vi "Control_Sensing_Sep.vi"() -> ()   [LabVIEW 2019]
uses:
  Control 1.ctl
  <vilib>/myRIO/Instrument Drivers/Onboard IO/I2C/typedefs/I2C User Configuration.ctl
  <vilib>/myRIO/Instrument Drivers/Onboard IO/I2C/typedefs/I2C Transfer Rate.ctl
  <vilib>/myRIO/Instrument Drivers/Onboard IO/I2C/typedefs/I2C Reference.ctl
  <vilib>/myRIO/Common/Instrument Driver Framework/Utilities/typedefs/myRIO Generic Hardware Reference.ctl
  <vilib>/myRIO/Common/Instrument Driver Framework/Utilities/typedefs/Hardware Version Enum.ctl
  <vilib>/myRIO/Common/Instrument Driver Framework/Utilities/typedefs/myRIO v1.0 Reference.ctl
  <vilib>/myRIO/Common/Instrument Driver Framework/Utilities/typedefs/Generic FPGA Reference.ctl
  <vilib>/myRIO/Common/Instrument Driver Framework/myRIO v1.0/I2C/typedefs/I2C Channels Enum.ctl
  <vilib>/myRIO/Instrument Drivers/Onboard IO/I2C/typedefs/I2C Configuration.ctl
  <vilib>/userDefined/High Color/nirio_resource_hc.ctl
  <vilib>/myRIO/Instrument Drivers/Onboard IO/AI/typedefs/AI Reference.ctl
  <vilib>/myRIO/Common/Instrument Driver Framework/myRIO v1.0/AI/typedefs/AI Channels List.ctl
  <vilib>/myRIO/Common/Instrument Driver Framework/myRIO v1.0/AI/typedefs/AI Channels Enum.ctl
  <vilib>/myRIO/Common/Instrument Driver Framework/Utilities/typedefs/Analog Scaling Constants List.ctl
  <vilib>/myRIO/Common/Instrument Driver Framework/Utilities/typedefs/Analog Scaling Constants.ctl
  <vilib>/myRIO/Instrument Drivers/Onboard IO/DIO/typedefs/DIO Reference.ctl
  <vilib>/myRIO/Common/Instrument Driver Framework/myRIO v1.0/DIO/typedefs/DIO Channels List.ctl
  <vilib>/myRIO/Common/Instrument Driver Framework/myRIO v1.0/DIO/typedefs/DIO Channels Enum.ctl
  <vilib>/myRIO/Instrument Drivers/Onboard IO/PWM/typedefs/PWM Reference.ctl
  <vilib>/myRIO/Common/Instrument Driver Framework/myRIO v1.0/PWM/typedefs/PWM Channels Enum.ctl
  <vilib>/myRIO/Instrument Drivers/Onboard IO/PWM/typedefs/PWM Configuration.ctl
  <vilib>/myRIO/Common/Instrument Driver Framework/Utilities/vis/Is FPGA Ref Available.vi
  <vilib>/myRIO/Common/Instrument Driver Framework/myRIO v1.0/I2C/vis/myRIO v1.1 Open I2C.vi
  <vilib>/myRIO/Instrument Drivers/Onboard IO/I2C/vis/Configure.vi
  <vilib>/myRIO/Instrument Drivers/Onboard IO/I2C/vis/Write.vi
  <vilib>/myRIO/Common/Instrument Driver Framework/myRIO v1.0/DIO/vis/myRIO v1.1 Open DIO.vi
  <vilib>/myRIO/Instrument Drivers/Onboard IO/DIO/vis/Read.vi
  <vilib>/myRIO/Common/Instrument Driver Framework/myRIO v1.0/AI/vis/myRIO v1.1 Open AI.vi
  <vilib>/myRIO/Instrument Drivers/Onboard IO/AI/vis/Read.vi
  <vilib>/myRIO/Instrument Drivers/Onboard IO/DIO/vis/Write.vi
  <vilib>/myRIO/Common/Instrument Driver Framework/myRIO v1.0/PWM/vis/myRIO v1.1 Open PWM.vi
  <vilib>/myRIO/Instrument Drivers/Onboard IO/PWM/vis/Set Duty Cycle and Frequency.vi
  <vilib>/myRIO/Instrument Drivers/Onboard IO/I2C/vis/Write Read.vi
  <vilib>/myRIO/Common/Instrument Driver Framework/myRIO v1.0/UART/vis/myRIO v1.0 Close UART.vi
  <vilib>/myRIO/Common/Instrument Driver Framework/Utilities/vis/Validate Channels.vi
  <vilib>/myRIO/Common/Instrument Driver Framework/myRIO v1.0/I2C/vis/myRIO v1.0 Reserve I2C.vi
  <vilib>/myRIO/Common/Instrument Driver Framework/myRIO v1.0/DIO/vis/myRIO v1.0 Reserve DIO.vi
  <vilib>/myRIO/Common/Instrument Driver Framework/myRIO v1.0/AI/vis/myRIO v1.0 Reserve AI.vi
  <vilib>/myRIO/Common/Instrument Driver Framework/myRIO v1.0/PWM/vis/myRIO v1.0 Reserve PWM.vi
  <vilib>/myRIO/Common/Instrument Driver Framework/myRIO v1.0/I2C/vis/myRIO v1.0 Build MUX Configuration I2C.vi
  <vilib>/myRIO/Common/Instrument Driver Framework/myRIO v1.0/Resource Manager/vis/myRIO v1.0 Reserve Channel List.vi
  <vilib>/myRIO/Common/Instrument Driver Framework/myRIO v1.0/DIO/vis/myRIO v1.0 Build MUX Configuration DIO.vi
  <vilib>/myRIO/Common/Instrument Driver Framework/myRIO v1.0/AI/vis/myRIO v1.0 Build MUX Configuration AI.vi
  <vilib>/myRIO/Common/Instrument Driver Framework/myRIO v1.0/PWM/vis/myRIO v1.0 Build MUX Configuration PWM.vi
  <vilib>/myRIO/Common/Instrument Driver Framework/myRIO v1.0/Resource Manager/vis/myRIO v1.0 Create Configuration List.vi
  <vilib>/myRIO/Common/Instrument Driver Framework/myRIO v1.0/Resource Manager/vis/myRIO v1.0 Reserve Channel.vi
  <vilib>/myRIO/Common/Instrument Driver Framework/myRIO v1.0/Resource Manager/vis/myRIO v1.0 Unreserve Channel.vi
  <vilib>/myRIO/Common/Instrument Driver Framework/myRIO v1.0/Resource Manager/vis/myRIO v1.0 Build Mutex Name.vi
  <vilib>/imath/engines/lvmath2/RunTimeEngine/NodeEndStatement/NIMS_NodeEndStatement_Output.vi
  <instcachedir>/0/NIMS_NodeEndStatement_Output_53EC0D466D134D7ABD903AC30B43404B.lvgen/NIMS_NodeEndStatement_Output_53EC0D466D134D7ABD903AC30B43404B_000.vi
  <instcachedir>/0/NIMS_NodeEndStatement_Output_53EC0D466D134D7ABD903AC30B43404B.lvgen/NIMS_NodeEndStatement_Output_53EC0D466D134D7ABD903AC30B43404B_005.vi
  <vilib>/imath/engines/lvmath2/RunTimeEngine/ErrorHandling/NIMS_Finalize Error.vi
  <vilib>/imath/engines/lvmath2/RunTimeEngine/BuiltInFunctions/length/NIMS_length(GV).vi
  <instcachedir>/0/NIMS_length(GV)_08A3D13377FD4E4B96F5795FBF3698FA.lvgen/NIMS_length(GV)_08A3D13377FD4E4B96F5795FBF3698FA_000.vi
  <vilib>/imath/engines/lvmath2/RunTimeEngine/BuiltInFunctions/ones/NIMS_V=ones(I32,I32).vi
  <vilib>/imathl/engines/lvmath/Functions/Error Handling/Create Error.vi
  <vilib>/imath/engines/lvmath2/RunTimeEngine/RangeToken/NIMS_Range.vi
  <instcachedir>/0/NIMS_Range_FADF6ADDA3E145BB934C8BD4C7DAAB97.lvgen/NIMS_Range_FADF6ADDA3E145BB934C8BD4C7DAAB97_000.vi
  <vilib>/imath/engines/lvmath2/RunTimeEngine/Managers/WorkSpace/UID Generator.vi
  <vilib>/imath/engines/lvmath2/RunTimeEngine/RunTimeType/NIMS_RunTimeType_From StrictType (excl LVString).vi
  <instcachedir>/0/NIMS_RunTimeType_From StrictType (excl LVString)_D8AFBA86A94845AAA577C895450664BD.lvgen/NIMS_RunTimeType_From StrictType (excl LVString)_D8AFBA86A94845AAA577C895450664BD_000.vi
  <vilib>/imath/engines/lvmath2/RunTimeEngine/LocalVariableDefStatement/MC_LocalVariableDefStatement_Display.vi
  <vilib>/imath/engines/lvmath2/RunTimeEngine/BuiltInFunctions/diag/NIMS_diag.vi
  <instcachedir>/0/NIMS_diag_DCAB8C8FDAF64F9E84492BB524435AA9.lvgen/NIMS_diag_DCAB8C8FDAF64F9E84492BB524435AA9_003.vi
  <vilib>/imath/engines/lvmath2/RunTimeEngine/BuiltInFunctions/mirrorh/NIMS_mirrorh(GM).vi
  <instcachedir>/0/NIMS_mirrorh(GM)_A650AD0D730A4A8EBE251B4C5C7CA115.lvgen/NIMS_mirrorh(GM)_A650AD0D730A4A8EBE251B4C5C7CA115_004.vi
  <vilib>/imath/engines/lvmath2/RunTimeEngine/RowToken/NIMS_RowToken_M_M.vi
  <instcachedir>/0/NIMS_RowToken_M_M_21FE36D058524603B8B587AC30FD72C2.lvgen/NIMS_RowToken_M_M_21FE36D058524603B8B587AC30FD72C2_005.vi
  <vilib>/imath/engines/lvmath2/RunTimeEngine/ErrorHandling/NIMS_Create Error From Enums.vi
  <vilib>/imath/engines/lvmath2/RunTimeEngine/Managers/SymbolTable/Clear UID.vi
  <instcachedir>/0/NIMS_NodeEndStatement_Output_53EC0D466D134D7ABD903AC30B43404B.lvgen/NIMS_NodeEndStatement_Output_53EC0D466D134D7ABD903AC30B43404B_002.vi
  <instcachedir>/0/NIMS_NodeEndStatement_Output_53EC0D466D134D7ABD903AC30B43404B.lvgen/NIMS_NodeEndStatement_Output_53EC0D466D134D7ABD903AC30B43404B_010.vi
  <vilib>/Utility/VariantDataType/GetNumericInfo.vi
  <vilib>/Utility/error.llb/Error Cluster From Error Code.vi
  <vilib>/myRIO/Common/Instrument Driver Framework/myRIO v1.0/myRIO v1.1 Open.vi
  <vilib>/myRIO/Common/Instrument Driver Framework/Utilities/vis/IO Manager.vi
  <vilib>/myRIO/Common/Instrument Driver Framework/Utilities/vis/Configuration Manager.vi
  <vilib>/myRIO/Common/Instrument Driver Framework/myRIO v1.0/Resource Manager/vis/myRIO v1.0 Configure IO.vi
  <vilib>/myRIO/Common/Instrument Driver Framework/myRIO v1.0/myRIO v1.0 Close.vi
  <vilib>/myRIO/Common/Instrument Driver Framework/myRIO v1.0/I2C/vis/myRIO v1.0 Configure I2C.vi
  <vilib>/myRIO/Common/Instrument Driver Framework/myRIO v1.0/I2C/vis/myRIO v1.0 Write I2C.vi
  <vilib>/myRIO/Common/Instrument Driver Framework/myRIO v1.0/AI/vis/myRIO v1.0 Get Scaling Constants AI.vi
  <vilib>/myRIO/Common/Instrument Driver Framework/myRIO v1.0/AI/vis/myRIO v1.0 Read AI.vi
  <vilib>/myRIO/Common/Instrument Driver Framework/myRIO v1.0/DIO/vis/myRIO v1.0 Read DIO.vi
  <vilib>/myRIO/Common/Instrument Driver Framework/myRIO v1.0/DIO/vis/myRIO v1.0 Write DIO.vi
  <vilib>/myRIO/Common/Instrument Driver Framework/myRIO v1.0/PWM/vis/myRIO v1.0 Write PWM.vi
  <vilib>/myRIO/Common/Instrument Driver Framework/myRIO v1.0/I2C/vis/myRIO v1.0 Read I2C.vi
  LabVIEW Data/MathScriptVIs/MCStatic_41946317732_dea1fbe93744f113d60bcd9143af88e2.vi
  <instcachedir>/0/MCStatic_41946317732_dea1fbe93744f113d60bcd9143af88e2_83BEAC789B7B43BC9406FCFCD10D71C6.lvgen/MCStatic_41946317732_dea1fbe93744f113d60bcd9143af88e2_83BEAC789B7B43BC9406FCFCD10D71C6_001.vi
  <vilib>/imath/engines/lvmath2/RunTimeEngine/ArithmeticOperatorToken/NIMS_ArithmeticOperator_multmx.vi
  <instcachedir>/0/NIMS_ArithmeticOperator_multmx_77F1D2D6F4D94BA7A97C4E7185C02392.lvgen/NIMS_ArithmeticOperator_multmx_77F1D2D6F4D94BA7A97C4E7185C02392_003.vi
  <instcachedir>/0/NIMS_diag_DCAB8C8FDAF64F9E84492BB524435AA9.lvgen/NIMS_diag_DCAB8C8FDAF64F9E84492BB524435AA9_002.vi
  <vilib>/imath/engines/lvmath2/RunTimeEngine/BuiltInFunctions/max/1 input/NIMS_max(CM).vi
  <instcachedir>/0/NIMS_max(CM)_ECFF9CEF2CF74B92B05BC258ECD38873.lvgen/NIMS_max(CM)_ECFF9CEF2CF74B92B05BC258ECD38873_000.vi
  <vilib>/imath/engines/lvmath/Functions/Error Handling/MergeErrorsWrapper.vi
  <vilib>/imath/engines/lvmath2/RunTimeEngine/CommandStatement/MC_CommandStatement_break.vi
  LabVIEW Data/MathScriptVIs/MCStatic_41946317732_a250ab093b6754267866aa6e19f5e231.vi
  <instcachedir>/0/MCStatic_41946317732_a250ab093b6754267866aa6e19f5e231_ACFC674F96FF402A8C91EA69A4079298.lvgen/MCStatic_41946317732_a250ab093b6754267866aa6e19f5e231_ACFC674F96FF402A8C91EA69A4079298_000.vi
  <vilib>/imath/engines/lvmath2/RunTimeEngine/ArithmeticOperatorToken/NIMS_ArithmeticOperator_minus.vi
  <instcachedir>/0/NIMS_ArithmeticOperator_minus_12BFF9710EA5430A9EE87C5BC3F65186.lvgen/NIMS_ArithmeticOperator_minus_12BFF9710EA5430A9EE87C5BC3F65186_009.vi
  <vilib>/imath/engines/lvmath2/RunTimeEngine/BuiltInFunctions/norm/NIMS_norm(GM,DBL).vi
  <instcachedir>/0/NIMS_norm(GM,DBL)_8BCB088F207E48DF95CF5C1DC502F84D.lvgen/NIMS_norm(GM,DBL)_8BCB088F207E48DF95CF5C1DC502F84D_001.vi
  <vilib>/imath/engines/lvmath2/RunTimeEngine/BuiltInFunctions/abs/NIMS_abs(signed).vi
  <instcachedir>/0/NIMS_abs(signed)_C4FCB8E6058B49B797C7C8D53CA5F6EC.lvgen/NIMS_abs(signed)_C4FCB8E6058B49B797C7C8D53CA5F6EC_003.vi
  <vilib>/imath/engines/lvmath2/RunTimeEngine/BuiltInFunctions/max/1 input/NIMS_max(RM).vi
  <instcachedir>/0/NIMS_max(RM)_0B4294876EE440609D638D7C5C6E788E.lvgen/NIMS_max(RM)_0B4294876EE440609D638D7C5C6E788E_000.vi
  <vilib>/imath/engines/lvmath2/RunTimeSupport/NIMS_Get Scalar_w Error.vi
  <instcachedir>/0/NIMS_Get Scalar_w Error_90FA09EFB1C84794B43793796939E0E3.lvgen/NIMS_Get Scalar_w Error_90FA09EFB1C84794B43793796939E0E3_010.vi
  <vilib>/imath/engines/lvmath2/RunTimeEngine/BuiltInFunctions/eye/NIMS_M=eye(I32).vi
  <instcachedir>/0/NIMS_ArithmeticOperator_multmx_77F1D2D6F4D94BA7A97C4E7185C02392.lvgen/NIMS_ArithmeticOperator_multmx_77F1D2D6F4D94BA7A97C4E7185C02392_007.vi
  <vilib>/imath/engines/lvmath2/RunTimeEngine/ArithmeticOperatorToken/NIMS_ArithmeticOperator_plus.vi
  <instcachedir>/0/NIMS_ArithmeticOperator_plus_5C9385B0197D46E2B844C41E02F9EC39.lvgen/NIMS_ArithmeticOperator_plus_5C9385B0197D46E2B844C41E02F9EC39_002.vi
  <vilib>/imath/engines/lvmath2/RunTimeEngine/ArithmeticOperatorToken/NIMS_ArithmeticOperator_leftdivmx(C,C).vi
  <instcachedir>/0/NIMS_ArithmeticOperator_leftdivmx(C,C)_FFA86DC98B994D28AA7593516F1DAFDA.lvgen/NIMS_ArithmeticOperator_leftdivmx(C,C)_FFA86DC98B994D28AA7593516F1DAFDA_000.vi
  <vilib>/imath/engines/lvmath2/RunTimeEngine/ArithmeticOperatorToken/NIMS_ArithmeticOperator_rightdiv.vi
  <instcachedir>/0/NIMS_ArithmeticOperator_rightdiv_23AAA10E4B1E4564B1AF1956090A34B0.lvgen/NIMS_ArithmeticOperator_rightdiv_23AAA10E4B1E4564B1AF1956090A34B0_004.vi
  <instcachedir>/0/NIMS_ArithmeticOperator_minus_12BFF9710EA5430A9EE87C5BC3F65186.lvgen/NIMS_ArithmeticOperator_minus_12BFF9710EA5430A9EE87C5BC3F65186_008.vi
  <vilib>/imath/engines/lvmath2/RunTimeEngine/ArithmeticOperatorToken/NIMS_ArithmeticOperator_rightdivmx(C,C).vi
  <instcachedir>/0/NIMS_ArithmeticOperator_rightdivmx(C,C)_4C9834AF73264B85B2EC0ABB36B07CCF.lvgen/NIMS_ArithmeticOperator_rightdivmx(C,C)_4C9834AF73264B85B2EC0ABB36B07CCF_000.vi
  <vilib>/imath/engines/lvmath2/RunTimeEngine/ArithmeticOperatorToken/NIMS_ArithmeticOperator_powermx(M,M).vi
  <vilib>/imath/engines/lvmath2/RunTimeEngine/BuiltInFunctions/max/2 inputs/NIMS_max(CG,CG)-no size check.vi
  <instcachedir>/0/NIMS_max(CG,CG)-no size check_0D8807EB624448B1961BA94FD6C7666D.lvgen/NIMS_max(CG,CG)-no size check_0D8807EB624448B1961BA94FD6C7666D_000.vi
  <instcachedir>/0/MCStatic_41946317732_dea1fbe93744f113d60bcd9143af88e2_83BEAC789B7B43BC9406FCFCD10D71C6.lvgen/MCStatic_41946317732_dea1fbe93744f113d60bcd9143af88e2_83BEAC789B7B43BC9406FCFCD10D71C6_000.vi
  <vilib>/imath/engines/lvmath2/RunTimeEngine/CommandStatement/NIMS_CommandStatement_MaskErr.vi
  <vilib>/imath/engines/lvmath2/RunTimeEngine/NodeEndStatement/NIMS_NodeEndStatement_Get Vector.vi
  <instcachedir>/0/NIMS_NodeEndStatement_Get Vector_92F29E6578CC4FEABDAC0B727A70E862.lvgen/NIMS_NodeEndStatement_Get Vector_92F29E6578CC4FEABDAC0B727A70E862_003.vi
  LabVIEW Data/MathScriptVIs/MCStatic_41946317732_9c6833b6fe53c90f9d53b911055dbc2d.vi
  <instcachedir>/0/MCStatic_41946317732_9c6833b6fe53c90f9d53b911055dbc2d_E61D551C9E9C456B8849957B0E9A24F9.lvgen/MCStatic_41946317732_9c6833b6fe53c90f9d53b911055dbc2d_E61D551C9E9C456B8849957B0E9A24F9_001.vi
  LabVIEW Data/MathScriptVIs/MCStatic_41946317732_9dae5a46252e3975b3d5cf9958ddddff.vi
  <instcachedir>/0/MCStatic_41946317732_9dae5a46252e3975b3d5cf9958ddddff_C527FE29D43C4C7A88FB384EB1727467.lvgen/MCStatic_41946317732_9dae5a46252e3975b3d5cf9958ddddff_C527FE29D43C4C7A88FB384EB1727467_000.vi
  <instcachedir>/0/MCStatic_41946317732_9c6833b6fe53c90f9d53b911055dbc2d_E61D551C9E9C456B8849957B0E9A24F9.lvgen/MCStatic_41946317732_9c6833b6fe53c90f9d53b911055dbc2d_E61D551C9E9C456B8849957B0E9A24F9_000.vi
  <vilib>/myRIO/Common/Instrument Driver Framework/Utilities/vis/FPGA Ref Manager.vi
  <vilib>/myRIO/Common/Instrument Driver Framework/myRIO v1.0/myRIO v1.0 Reset FPGA.vi
  <vilib>/myRIO/Common/Instrument Driver Framework/myRIO v1.0/IRQ/vis/myRIO v1.0 IRQ Info FGV.vi
  <vilib>/myRIO/Common/Instrument Driver Framework/myRIO v1.0/IRQ/vis/myRIO v1.0 Timer IRQ Info FGV.vi
  <vilib>/myRIO/Common/Instrument Driver Framework/myRIO v1.0/IRQ/vis/myRIO v1.0 ISR Agent.vi
  <vilib>/myRIO/Instrument Drivers/Utilities/vis/Reset Index.vi
  <vilib>/myRIO/Common/Instrument Driver Framework/myRIO v1.0/Resource Manager/vis/myRIO v1.0 Block Write Resource Manager.vi
  <vilib>/myRIO/Express VI/Onboard IO/I2C/I2C Express VI.xnode
  <vilib>/myRIO/Instrument Drivers/Onboard IO/I2C/vis/myRIO I2C Open.xnode
  <vilib>/myRIO/Express VI/Onboard IO/AI/AI Express VI.xnode
  <vilib>/myRIO/Instrument Drivers/Onboard IO/AI/vis/myRIO AI Open.xnode
  <vilib>/myRIO/Express VI/Onboard IO/DI/DI Express VI.xnode
  <vilib>/myRIO/Instrument Drivers/Onboard IO/DIO/vis/myRIO DIO Open.xnode
  <vilib>/myRIO/Express VI/Onboard IO/DO/DO Express VI.xnode
  <vilib>/myRIO/Express VI/Onboard IO/PWM/PWM Express VI.xnode
  <vilib>/myRIO/Instrument Drivers/Onboard IO/PWM/vis/myRIO PWM Open.xnode
  magnetic_sensing-main/Analytic_Jacobian_Mag_cir_array_noM.m
  magnetic_sensing-main/PM_forward_field_noM.m
  magnetic_sensing-main/Analytic_Jacobian_Mag_cir_array_test.m
  magnetic_sensing-main/PM_forward_field.m
  <vilib>/myRIO/Instrument Drivers/Onboard IO/I2C/I2C.lvlib
  <vilib>/myRIO/Instrument Drivers/Utilities/Utilities.lvlib
  <vilib>/myRIO/Instrument Drivers/Onboard IO/PWM/PWM.lvlib
  <vilib>/myRIO/Instrument Drivers/Onboard IO/DIO/DIO.lvlib
  <vilib>/imath/engines/lvmath2/RunTimeEngine/Managers/SymbolTable/NIMS_WorkSpace.lvlib
  <instcachedir>/0/MCStatic_41946317732_a250ab093b6754267866aa6e19f5e231_ACFC674F96FF402A8C91EA69A4079298.lvgen/MCStatic_41946317732_a250ab093b6754267866aa6e19f5e231_ACFC674F96FF402A8C91EA69A4079298_001.vi
  <instcachedir>/0/MCStatic_41946317732_9dae5a46252e3975b3d5cf9958ddddff_C527FE29D43C4C7A88FB384EB1727467.lvgen/MCStatic_41946317732_9dae5a46252e3975b3d5cf9958ddddff_C527FE29D43C4C7A88FB384EB1727467_001.vi
  <vilib>/myRIO/Instrument Drivers/Onboard IO/AI/AI.lvlib
panel:
  out "Duty Ratio":dbl
  in  "Steering gain":dbl=1.0
  out "Encoder 2":dbl(graph)
  out "Sensing time":u32
  in  "Bifur?":bool
  in  "M":dbl
  in  "Update M in realtime?":bool
  in  "Clear plot?":bool
  out "pm_hat_opt":dbl[](array[numeric])
  in  "stop":bool
  in  "Actuation on?":bool
  in  "Action Mode":T1=enum."Sensing"
  out "XY Graph":cluster{dbl[], dbl[]}[](graph)
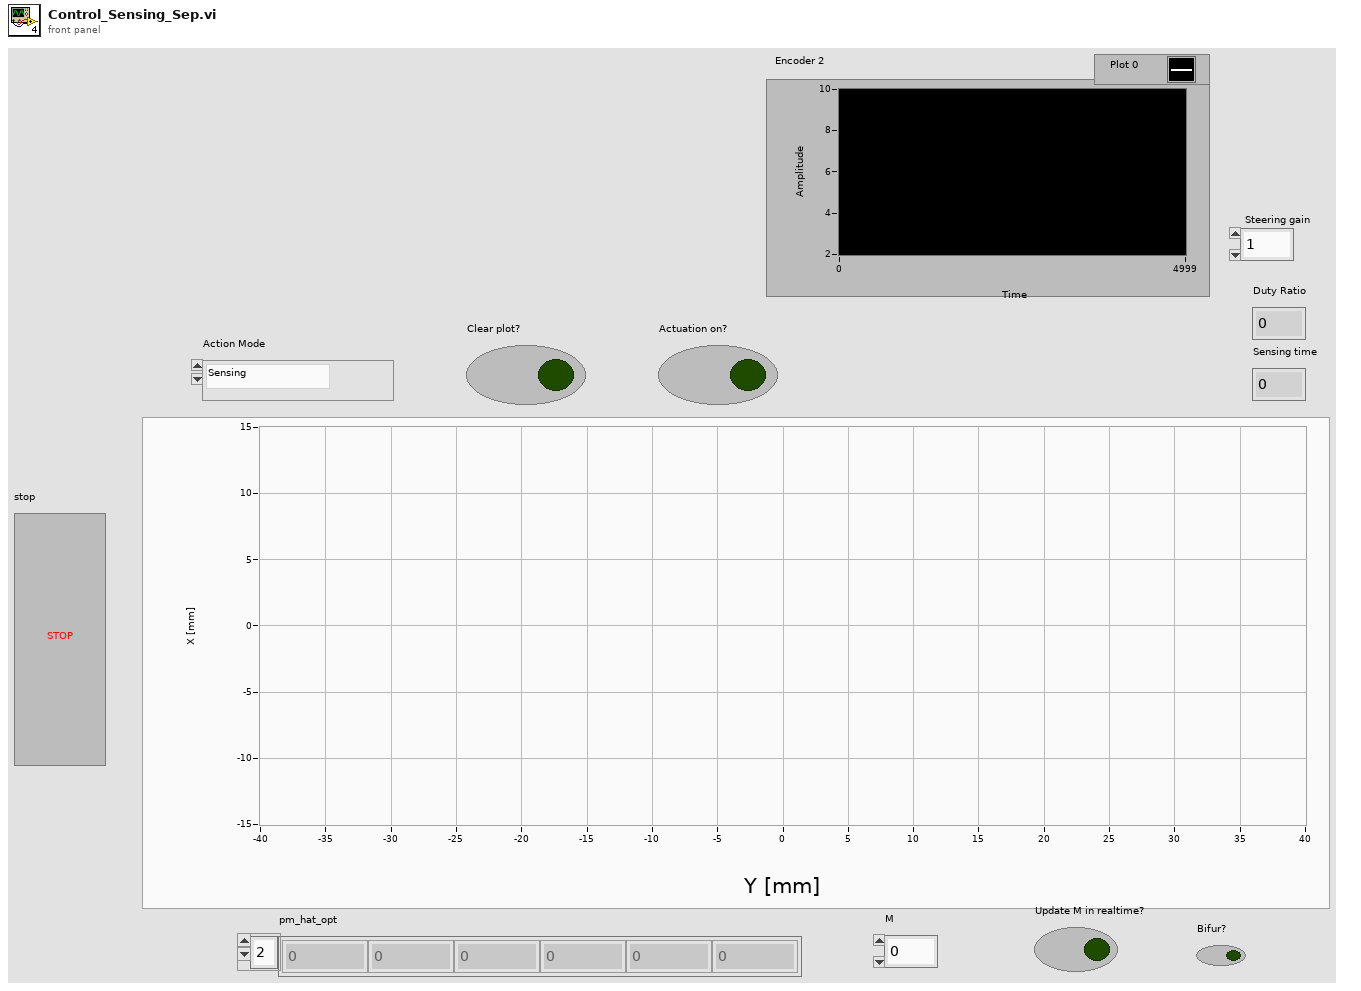
[diagram p1: front panel]
types:
  T1 = typedef "Control 1.ctl" = enum16{"Actuation", "Waiting", "Sensing"}
  T2 = typedef "I2C.lvlib/I2C Reference.ctl" = cluster{"myRIO Reference":T3, "I2C Channels Enum":T7, "I2C Configuration":T8}
  T3 = typedef "myRIO Generic Hardware Reference.ctl" = cluster{"myRIO Model":T4, "myRIO Hardware Reference":T5}
  T4 = typedef "Hardware Version Enum.ctl" = enum16{"Unknown", "myRIO-1900", "myRIO-1950", "roboRIO", "NI ELVIS RIO CM", "ELVIS III"}
  T5 = typedef "myRIO v1.0 Reference.ctl" = cluster{"Generic FPGA Reference":T6, "Allow multiple opens":bool}
  T6 = typedef "Generic FPGA Reference.ctl" = refnum<k20>
  T7 = typedef "I2C Channels Enum.ctl" = enum16{"Not Connected", "A/I2C", "B/I2C", "I2C/I2C"}
  T8 = typedef "I2C.lvlib/I2C Configuration.ctl" = cluster{"I2C Transfer Rate":T9}
  T9 = typedef "I2C.lvlib/I2C Transfer Rate.ctl" = enum16{"Standard mode (100 kbps)", "Fast mode (400 kbps)"}
  T10 = typedef "I2C.lvlib/I2C User Configuration.ctl" = cluster{"I2C Transfer Rate":T9}
  T11 = typedef "nirio_resource_hc.ctl" = tag
  T12 = typedef "DIO.lvlib/DIO Reference.ctl" = cluster{"myRIO Reference":T3, "DIO Channels List":T13}
  T13 = typedef "DIO Channels List.ctl" = T14[]
  T14 = typedef "DIO Channels Enum.ctl" = enum16{"Not Connected", "C/DIO0", "C/DIO1", "C/DIO2", "C/DIO3", "C/DIO4", "C/DIO5", "C/DIO6", "C/DIO7", "A/DIO0", "A/DIO1", "A/DIO2", "A/DIO3", "A/DIO4", "A/DIO5", "A/DIO6", "A/DIO7", "A/DIO8", "A/DIO9", "A/DIO10", "A/DIO11", "A/DIO12", "A/DIO13", "A/DIO14", "A/DIO15", "A/DIO16", "A/DIO17", "A/DIO18", "A/DIO19", "B/DIO0", "B/DIO1", "B/DIO2", "B/DIO3", "B/DIO4", "B/DIO5", "B/DIO6", "B/DIO7", "B/DIO8", "B/DIO9", "B/DIO10", "B/DIO11", "B/DIO12", "B/DIO13", "B/DIO14", "B/DIO15", "B/DIO16", "B/DIO17", "B/DIO18", "B/DIO19", "LED0", "LED1", "LED2", "LED3", "Button0", "DIO/DIO0", "DIO/DIO1", "DIO/DIO2", "DIO/DIO3", "DIO/DIO4", "DIO/DIO5", "DIO/DIO6", "DIO/DIO7", "DIO/DIO8", "DIO/DIO9", "SPI/CS0", "SPI/CS1", "SPI/CS2", "SPI/CS3", "LED RADIO (Green)", "LED RADIO (Red)", "LED COMM (Green)", "LED COMM (Red)", "LED MODE (Green)", "LED MODE (Red)"}
  T15 = typedef "AI.lvlib/AI Reference.ctl" = cluster{"myRIO Reference":T3, "AI Channels List":T16, "AI Scaling Constants List":T18}
  T16 = typedef "AI Channels List.ctl" = T17[]
  T17 = typedef "AI Channels Enum.ctl" = enum16{"Not Connected", "AudioIn/Left", "AudioIn/Right", "C/AI0", "C/AI1", "A/AI0", "A/AI1", "A/AI2", "A/AI3", "A/AI4", "A/AI5", "A/AI6", "A/AI7", "B/AI0", "B/AI1", "B/AI2", "B/AI3", "B/AI4", "B/AI5", "B/AI6", "B/AI7", "AI/AI0", "AI/AI1", "AI/AI2", "AI/AI3", "A/AI0 (DIFF)", "A/AI1 (DIFF)", "A/AI2 (DIFF)", "A/AI3 (DIFF)", "B/AI0 (DIFF)", "B/AI1 (DIFF)", "B/AI2 (DIFF)", "B/AI3 (DIFF)"}
  T18 = typedef "Analog Scaling Constants List.ctl" = T19[]
  T19 = typedef "Analog Scaling Constants.ctl" = cluster{"LSB Weight (Volts)":dbl, "Offset (Volts)":dbl, "Signed?":bool}
  T20 = typedef "PWM.lvlib/PWM Reference.ctl" = cluster{"myRIO Reference":T3, "PWM Channels Enum":T21, "PWM Configuration":T22}
  T21 = typedef "PWM Channels Enum.ctl" = enum16{"Not Connected", "C/PWM0", "C/PWM1", "A/PWM0", "A/PWM1", "A/PWM2", "A/PWM3", "A/PWM4", "A/PWM5", "A/PWM6", "A/PWM7", "A/PWM8", "A/PWM9", "A/PWM10", "A/PWM11", "A/PWM12", "A/PWM13", "A/PWM14", "A/PWM15", "A/PWM16", "A/PWM17", "A/PWM18", "A/PWM19", "B/PWM0", "B/PWM1", "B/PWM2", "B/PWM3", "B/PWM4", "B/PWM5", "B/PWM6", "B/PWM7", "B/PWM8", "B/PWM9", "B/PWM10", "B/PWM11", "B/PWM12", "B/PWM13", "B/PWM14", "B/PWM15", "B/PWM16", "B/PWM17", "B/PWM18", "B/PWM19", "PWM/PWM0", "PWM/PWM1", "PWM/PWM2", "PWM/PWM3", "PWM/PWM4", "PWM/PWM5", "PWM/PWM6", "PWM/PWM7", "PWM/PWM8", "PWM/PWM9"}
  T22 = typedef "PWM.lvlib/PWM Configuration.ctl" = cluster{"Frequency":dbl, "Duty Cycle":dbl}
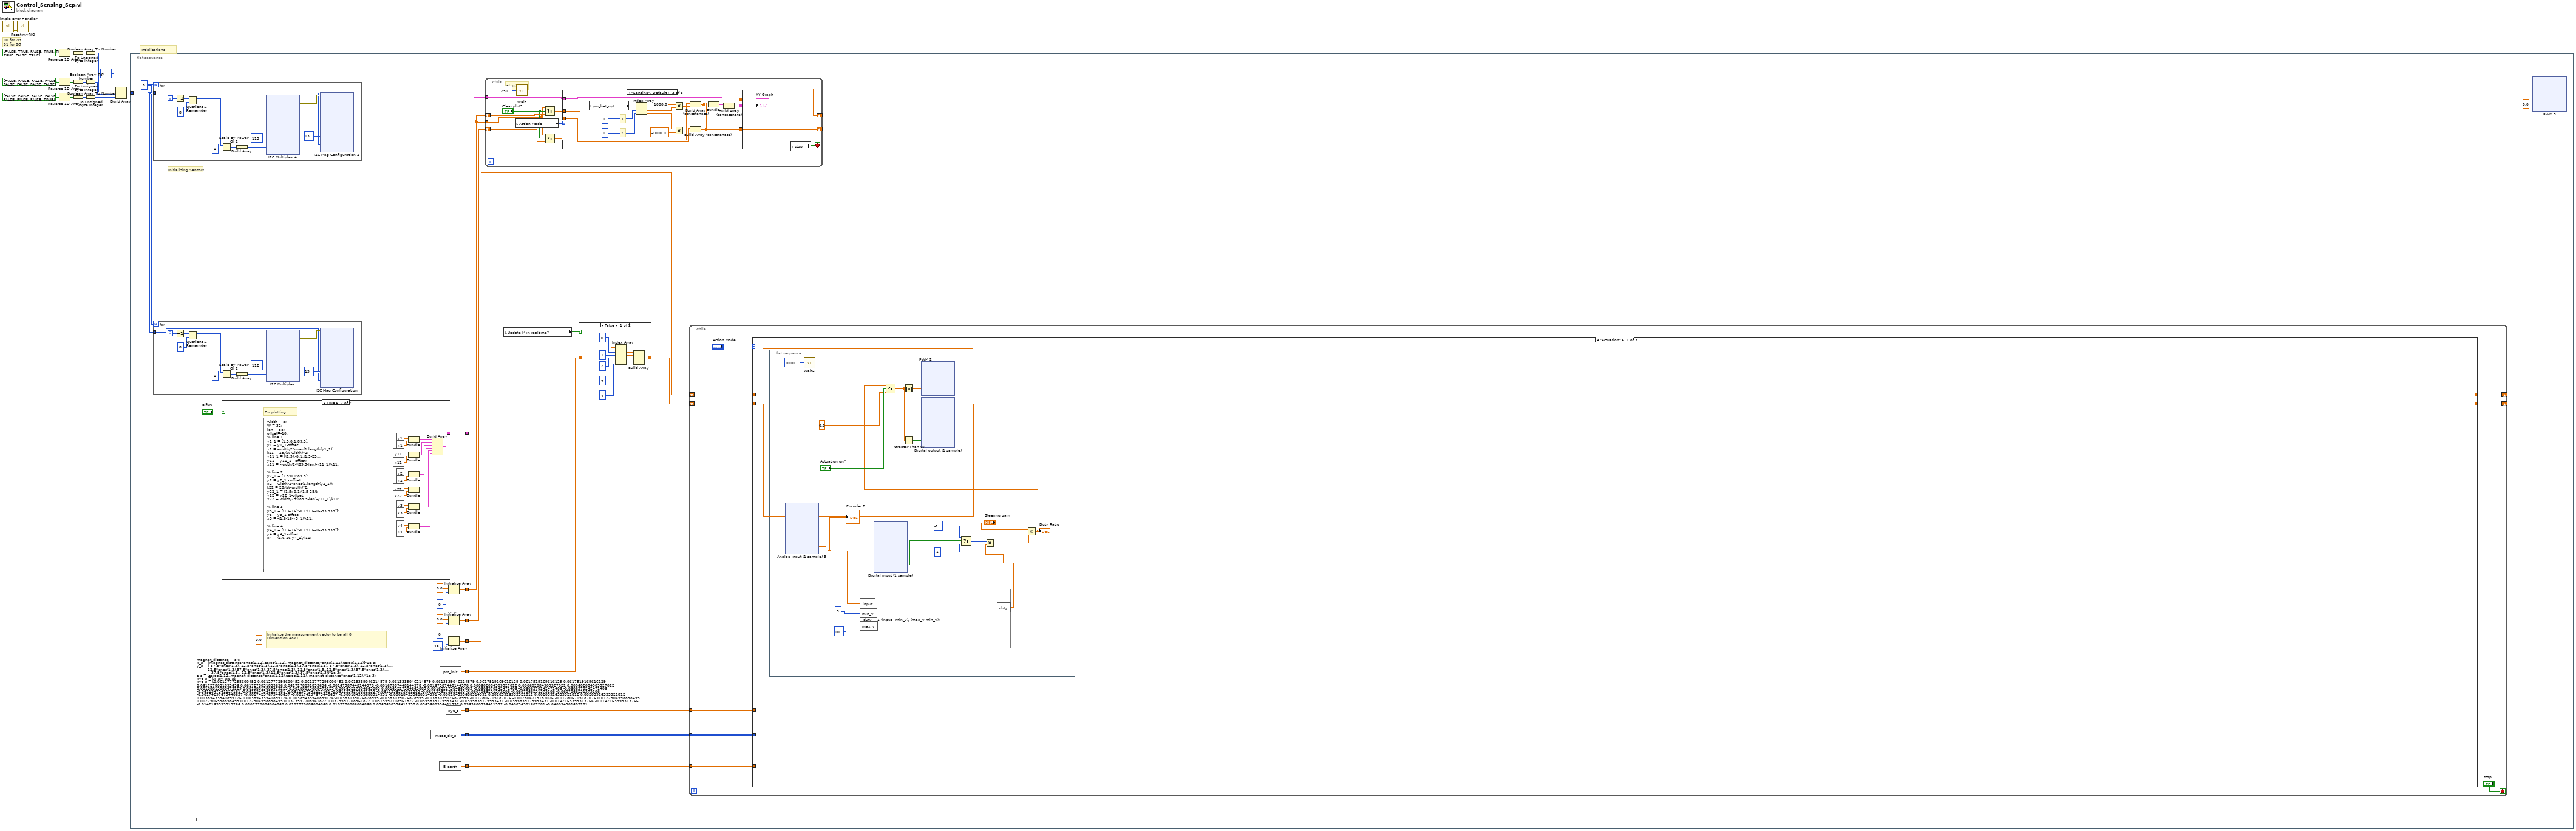
[diagram p0: block diagram]
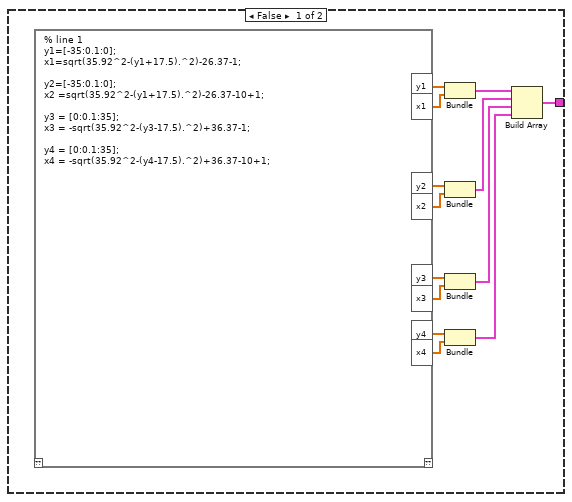
[diagram p2: hidden frame]
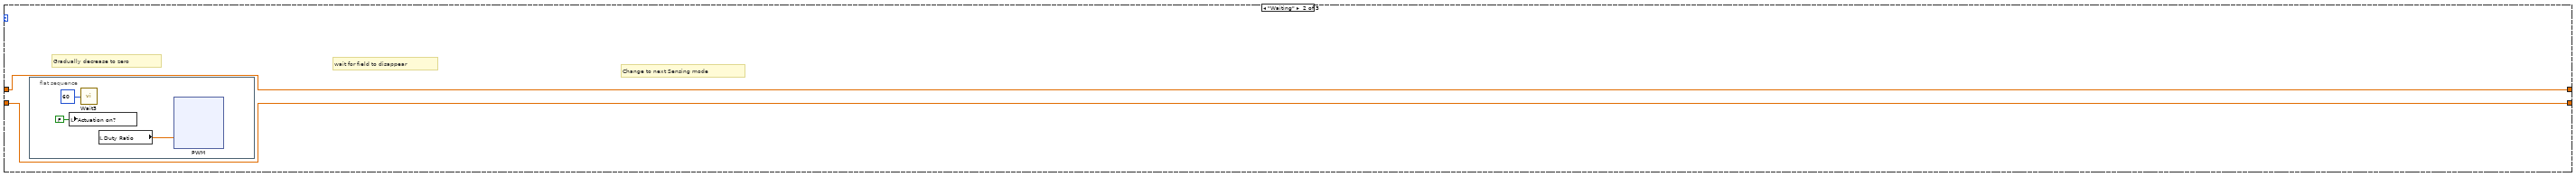
[diagram p4: hidden frame]
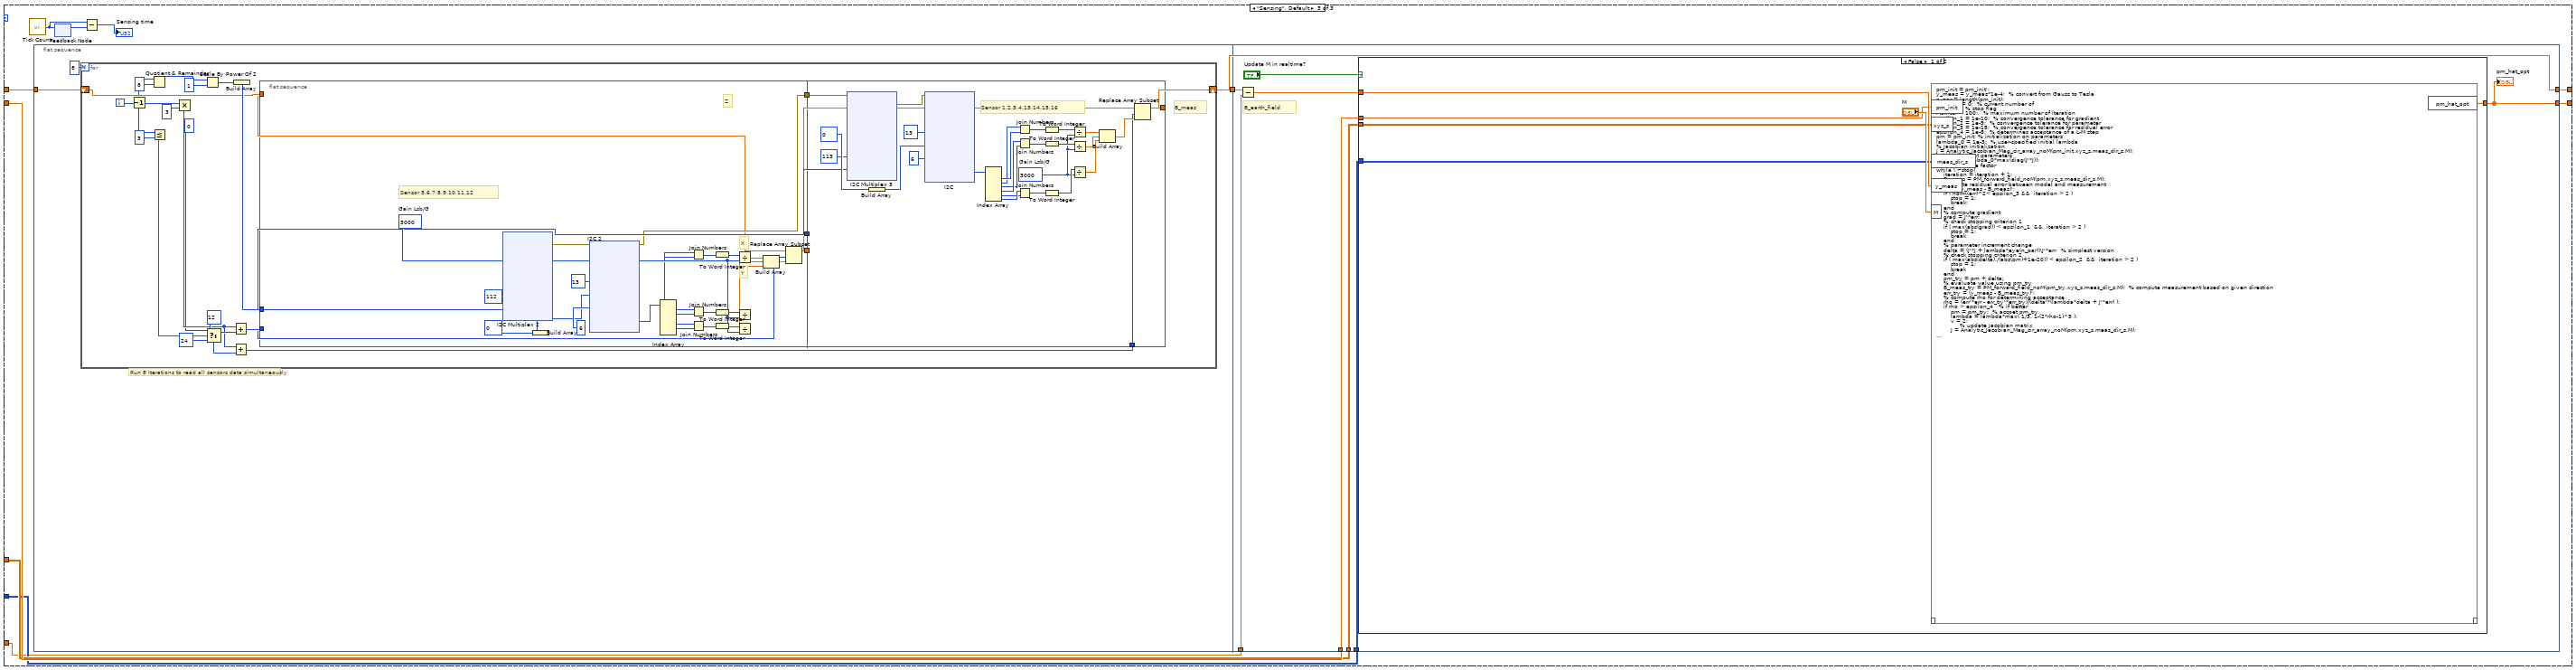
[diagram p5: hidden frame]
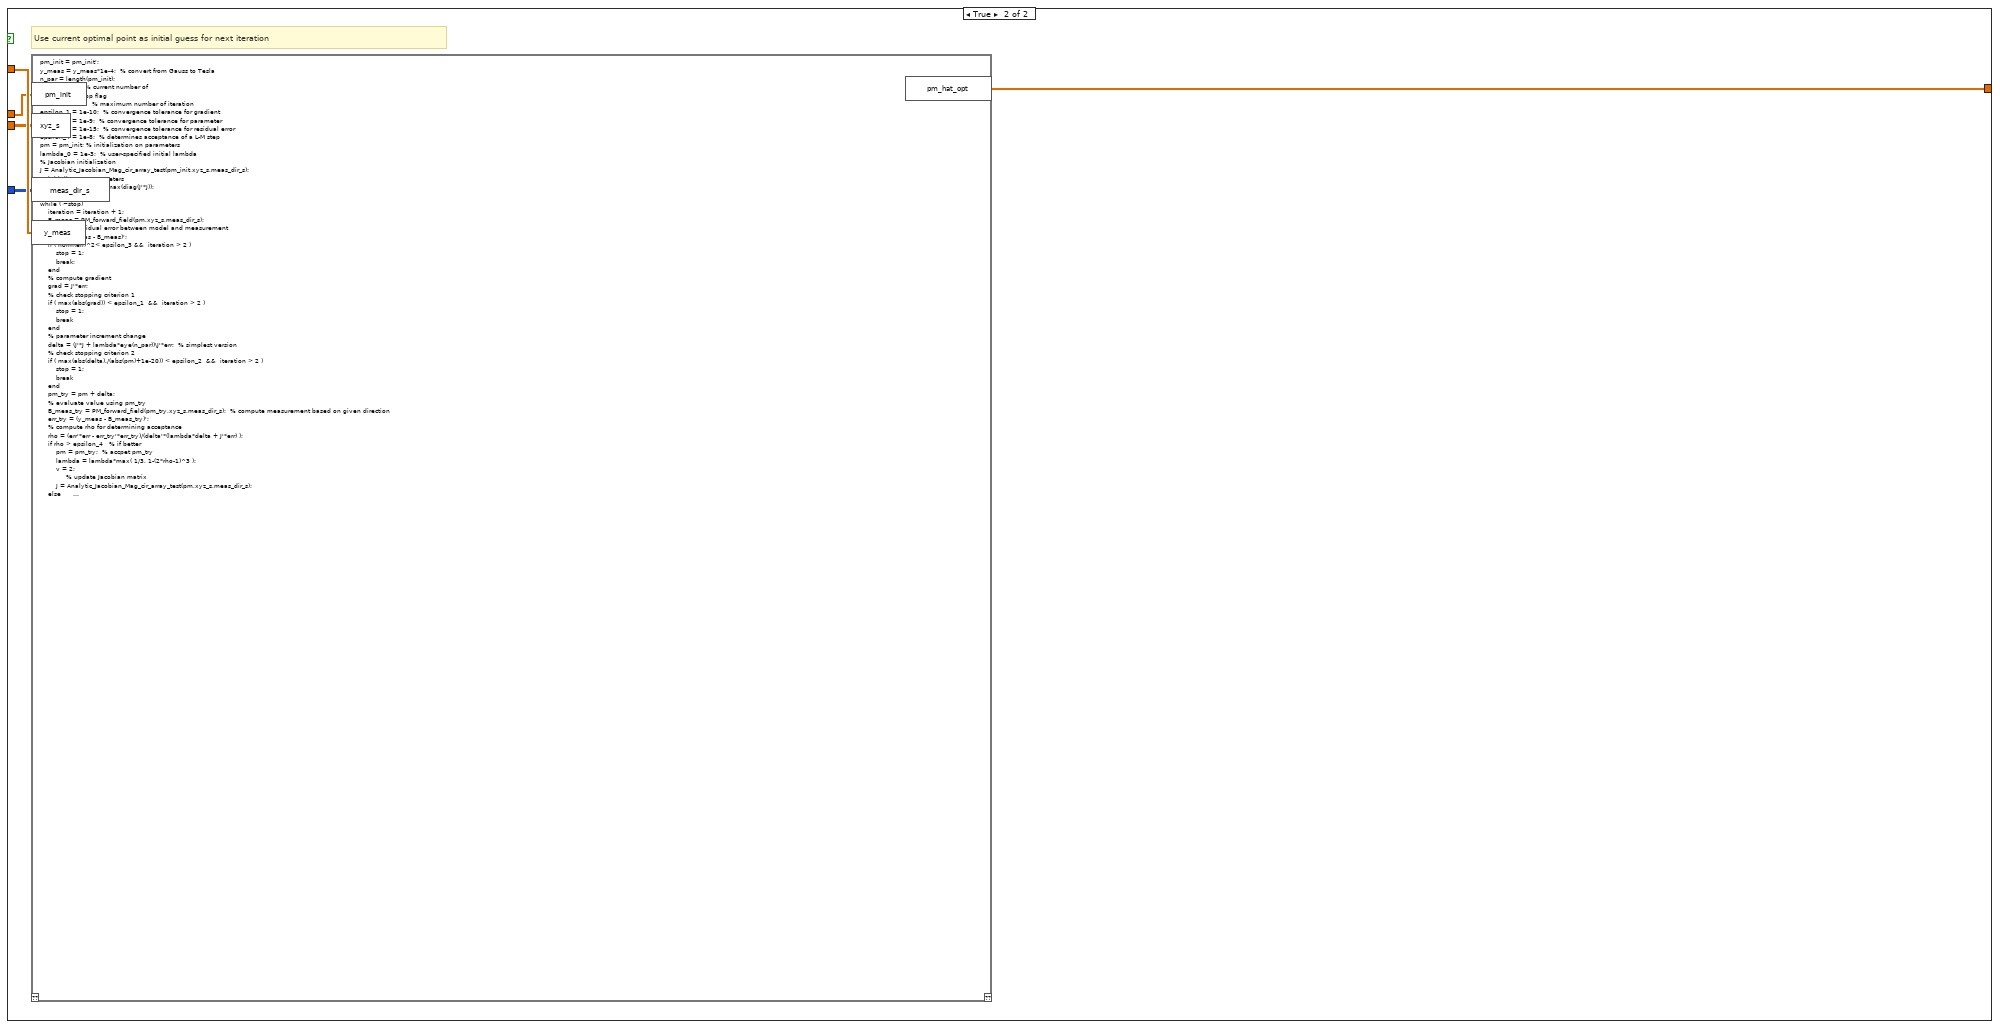
[diagram p6: hidden frame]
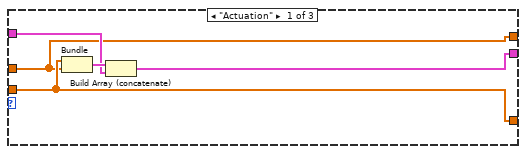
[diagram p7: hidden frame]
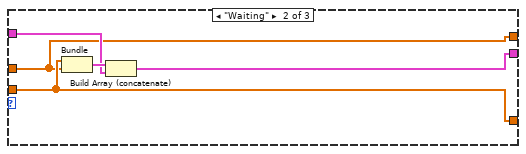
[diagram p8: hidden frame]
diagram:
  # "Intializations"
  # "00 for 2G\n01 for 8G"
  n1 = call <vilib>:"Simple Error Handler.vi"() -> ("error out"=w4:errorcluster)  [unwired: 5 in, 4 out]
  n2 = call <vilib>:"Reset myRIO.vi"("error in (no error)"=w4) -> ()  [unwired: 10 in, 1 out]
  n3 = Reverse 1D Array(array=bool[] [FALSE, TRUE, FALSE, TRUE, TRUE, TRUE, FALSE, TRUE]) -> (reversed array=w17:bool[])
  n4 = Reverse 1D Array(array=bool[] [FALSE, FALSE, FALSE, FALSE, FALSE, FALSE, FALSE, FALSE]) -> (reversed array=w16:bool[])
  n5 = Reverse 1D Array(array=bool[] [FALSE, FALSE, FALSE, FALSE, FALSE, FALSE, FALSE, TRUE]) -> (reversed array=w14:bool[])
  n6 = Boolean Array To Number(Boolean array=w17) -> (number=w11:u32)
  n7 = Boolean Array To Number(Boolean array=w16) -> (number=w10:u32)
  n8 = Boolean Array To Number(Boolean array=w14) -> (number=w9:u32)
  n9 = To Unsigned Byte Integer(number=w11) -> (unsigned 8bit integer=w8:u8)
  n10 = To Unsigned Byte Integer(number=w10) -> (unsigned 8bit integer=w7:u8)
  n11 = To Unsigned Byte Integer(number=w9) -> (unsigned 8bit integer=w6:u8)
  n12 = Build Array(u8 9 ("address"), w8, w7, w6) -> (w5:u8[])
  n13 = flat-sequence {
    tunnel: w5 -> [w40]
    tunnel: [w38] -> w23
    tunnel: [w37] -> w22
    tunnel: [w34] -> w21
    tunnel: [w33] -> w20
    tunnel: [w32] -> w19
    tunnel: [w27] -> w3
    tunnel: [w26] -> w2
    tunnel: [w25] -> w1
    tunnel: w23 -> [w995]
    tunnel: w22 -> [w996]
    tunnel: w21 -> [w997]
    tunnel: w20 -> [w990]
    tunnel: w19 -> [w994]
    tunnel: w3 -> [w993]
    tunnel: w2 -> [w991]
    tunnel: w1 -> [w992]
    frame #0 {
      w39 = 8
      # "Initialize the measurement vector to be all 0\nDimension 48x1"
      # "Initializing Sensors"
      n14 = for {
        N: w39 -> [_]
        tunnel: w40 -> [w821]
        i -> [w815]
        n15 = Decrement(x=w815) -> (x-1=w814:i32)
        n16 = Quotient & Remainder(x=w814, y=8) -> (x-y*floor(x/y)=w816:i32)  [unwired: 1 out]
        n17 = Scale By Power Of 2(n=w816, x=1) -> (x*2^n=w818:i32)
        n18 = Build Array(w818) -> (w824:i32[])
        n19 = xnode "I2C Multiplex 4"("Slave Address (7-bit)"=u8 113, "Bytes to Write"=w824) -> ("error out"=w823:errorcluster)  [unwired: 1 in]
        n20 = xnode "I2C Mag Configuration 2"("Slave Address (7-bit)"=u8 13, "Bytes to Write"=w821, "error in (no error)"=w823) -> ()  [unwired: 1 out]
      }
      n21 = for {
        N: w39 -> [_]
        tunnel: w40 -> [w908]
        i -> [w902]
        n22 = Decrement(x=w902) -> (x-1=w901:i32)
        n23 = Quotient & Remainder(x=w901, y=8) -> (x-y*floor(x/y)=w903:i32)  [unwired: 1 out]
        n24 = Scale By Power Of 2(n=w903, x=1) -> (x*2^n=w905:i32)
        n25 = Build Array(w905) -> (w911:i32[])
        n26 = xnode "I2C Multiplex"("Slave Address (7-bit)"=u8 112, "Bytes to Write"=w911) -> ("error out"=w910:errorcluster)  [unwired: 1 in]
        n27 = xnode "I2C Mag Configuration"("Slave Address (7-bit)"=u8 13, "Bytes to Write"=w908, "error in (no error)"=w910) -> ()  [unwired: 1 out]
      }
      n28 = mathscript code="magnet_distance = 54;\nx_s = [magnet_distance*ones(1,12),zeros(1,12),-magnet_distance*ones(1,12),zeros(1,12)]*1e-3; \ny_s = [-37.5*ones(1,3),-12.5*ones(1,3),12.5*ones(1,3),37.5*ones(1,3),-37.5*ones(1,3),-12.5*ones(1,3),...\n         12.5*ones(1,3),37.5*ones(1,3),-37.5*ones(1,3),-12.5*ones(1,3),12.5*ones(1,3),37.5*ones(1,3),...\n           -37.5*ones(1,3),-12.5*ones(1,3),12.5*ones(1,3),37.5*ones(1,3)]*1e-3; \nz_s = [zeros(1,12),magnet_distance*ones(1,12),zeros(1,12),-magnet_distance*ones(1,12)]*1e-3; \nxyz_s = [x_s;y_s;z_s];  \nxyz_s = [0.0612777298600452 0.0612777298600452 0.0612777298600452 0.0613339046214879 0.0613339046214879 0.0613339046214879 0.0617519169616129 0.0617519169616129 0.0617519169616129 0.0617278031895696 0.0617278031895696 0.0617278031895696 -0.00167587448144978 -0.00167587448144978 -0.00167587448144978 0.000602084909327022 0.000602084909327022 0.000602084909327022 0.00188819008475229 0.00188819008475229 0.00188819008475229 0.00165227304665085 0.00165227304665085 0.00165227304665085 -0.0606370242471406 -0.0606370242471406 -0.0606370242471406 -0.0611347541127161 -0.0611347541127161 -0.0611347541127161 -0.0611396275851359 -0.0611396275851359 -0.0611396275851359 -0.0607066251575206 -0.0607066251575206 -0.0607066251575206 -0.00174297673440637 -0.00174297673440637 -0.00174297673440637 -0.000184533688514991 -0.000184533688514991 -0.000184533688514991 0.00203926333921812 0.00203926333921812 0.00203926333921812 0.00389433540899126 0.00389433540899126 0.00389433540899126;-0.0383039026828955 -0.0383039026828955 -0.0383039026828955 -0.012806715187076 -0.012806715187076 -0.012806715187076 0.0122506598898495 0.0122506598898495 0.0122506598898495 0.0373597708961822 0.0373597708961822 0.0373597708961822 -0.0395839775993431 -0.0395839775993431 -0.0395839775993431 -0.0142163399313766 -0.0142163399313766 -0.0142163399313766 0.0107770086004868 0.0107770086004868 0.0107770086004868 0.0365600556411557 0.0365600556411557 0.0365600556411557 -0.040094901607281 -0.040094901607281 -0.040094901607281 -0.0149090266343068 -0.0149090266343068 -0.0149090266343068 0.0107078118967093 0.0107078118967093 0.0107078118967093 0.0356978973873521 0.0356978973873521 0.0356978973873521 -0.0392056799428433 -0.0392056799428433 -0.0392056799428433 -0.0139322320487061 -0.0139322320487061 -0.0139322320487061 0.0112429513248133 0.0112429513248133 0.0112429513248133 0.0361205812401305 0.0361205812401305 0.0361205812401305;0.00307213814961651 0.00307213814961651 0.00307213814961651 0.0033242461093476 0.0033242461093476 0.0033242461093476 0.00389293419390068 0.00389293419390068 0.00389293419390068 0.00390199978115286 0.00390199978115286 0.00390199978115286 0.0640688323293379 0.0640688323293379 0.0640688323293379 0.0636929900573754 0.0636929900573754 0.0636929900573754 0.0635181326061399 0.0635181326061399 0.0635181326061399 0.0633759954094267 0.0633759954094267 0.0633759954094267 -0.00381527257187291 -0.00381527257187291 -0.00381527257187291 -0.00312975643341264 -0.00312975643341264 -0.00312975643341264 -0.00272771938684928 -0.00272771938684928 -0.00272771938684928 -0.00268843620404175 -0.00268843620404175 -0.00268843620404175 -0.0628805002941716 -0.0628805002941716 -0.0628805002941716 -0.063138590462401 -0.063138590462401 -0.063138590462401 -0.063695098330538 -0.063695098330538 -0.063695098330538 -0.0638823957044235 -0.0638823957044235 -0.0638823957044235]\nmeas_dir_s = [mirrorh(diag([1;-1;1])),...\n              mirrorh(diag([1;-1;1])),...\n              mirrorh(diag([1;-1;1])),...\n              mirrorh(diag([1;-1;1])),...\n              diag([-1;-1;1]),...\n              diag([-1;-1;1]),...\n              diag([-1;-1;1]),...\n              diag([-1;-1;1]),...\n              mirrorh(diag([-1;-1;-1])),...\n              mirrorh(diag([-1;-1;-1])),...\n              mirrorh(diag([-1;-1;-1])),...\n              mirrorh(diag([-1;-1;-1])),... \n              diag([1;-1;-1]),...\n              diag([1;-1;-1]),...\n              diag([1;-1;-1]),...\n              diag([1;-1;-1])];\npm_init = [0;0;0;pi/2;-pi/2;0.04];\nB_earth = [-0.553111111\t-0.374555556\t-0.122619048...\n-0.515809524\t-0.295809524\t-0.077047619...\n-0.636904762\t-0.354634921\t-0.125174603...\n-0.544126984\t-0.318142857\t-0.118666667...\n0.235396825\t-0.012873016\t-0.451079365...\n0.087587302\t-0.320460317\t-0.478063492...\n0.075079365\t-0.297063492\t-0.457571429...\n0.078126984\t-0.341047619\t-0.499793651...\n0.401380952\t-0.248206349\t0.061952381...\n0.469435484\t-0.180274194\t0.06766129...\n0.442419355\t-0.269870968\t0.077758065...\n0.489177419\t-0.270806452\t-0.108483871...\n0.009730159\t-0.086761905\t0.67131746...\n-0.059096774\t-0.115145161\t0.576403226...\n-0.076854839\t-0.088258065\t0.584709677...\n-0.100354839\t-0.071241935\t0.519322581]';\nB_earth = [-0.567333\t\t-0.364333\t\t-0.155...\n-0.535667\t-0.278667\t\t-0.131...\n-0.669\t\t-0.355333\t\t-0.165...\n-0.562\t\t-0.300667\t\t-0.163667...\n0.278333\t-0.006\t\t-0.464333...\n0.126667\t-0.311\t\t-0.51...\n0.117667\t-0.29\t\t-0.499333...\n0.116\t\t-0.326667\t\t-0.534333...\n0.468667\t-0.243667\t\t0.04...\n0.506667\t-0.171667\t\t0.116...\n0.476\t\t-0.279333\t\t0.0543333...\n0.538667\t-0.255\t\t-0.0236667...\n-0.0566667\t-0.0843333\t\t0.678667...\n-0.126667\t-0.107667\t\t0.598333...\n-0.147333\t-0.0766667\t\t0.605...\n-0.172333\t-0.0466667\t\t0.542]';"() -> ("meas_dir_s"=w38:i32[][], "xyz_s"=w37:dbl[][], "pm_init"=w33:dbl[], "B_earth"=w32:dbl[])  [unwired: 1 in, 1 out]
      n29 = case shown="True" "Bifur?" {
        tunnel: [w41 w180] -> w27
        frame False {
          n30 = mathscript code="% line 1\ny1=[-35:0.1:0];\nx1=sqrt(35.92^2-(y1+17.5).^2)-26.37-1;\n\ny2=[-35:0.1:0];\nx2 =sqrt(35.92^2-(y1+17.5).^2)-26.37-10+1;\n\ny3 = [0:0.1:35];\nx3 = -sqrt(35.92^2-(y3-17.5).^2)+36.37-1;\n\ny4 = [0:0.1:35];\nx4 = -sqrt(35.92^2-(y4-17.5).^2)+36.37-10+1;"() -> ("y1"=w53:dbl[], "x1"=w52:cdb[], "y2"=w50:dbl[], "x2"=w49:cdb[], "y3"=w48:dbl[], "x3"=w47:cdb[], "y4"=w46:dbl[], "x4"=w45:cdb[])  [unwired: 1 in, 1 out]
          n31 = Bundle("y1"=w53, "x1"=w52) -> (w51:cluster{"y1":dbl[], "x1":cdb[]})  [unwired: 1 in]
          n32 = Bundle("y2"=w50, "x2"=w49) -> (w44:cluster{"y2":dbl[], "x2":cdb[]})  [unwired: 1 in]
          n33 = Bundle("y3"=w48, "x3"=w47) -> (w43:cluster{"y3":dbl[], "x3":cdb[]})  [unwired: 1 in]
          n34 = Bundle("y4"=w46, "x4"=w45) -> (w42:cluster{"y4":dbl[], "x4":cdb[]})  [unwired: 1 in]
          n35 = Build Array(w51, w44, w43, w42) -> (w41:cluster{"y4":dbl[], "x4":cdb[]}[])
        }
        frame True {
          # "For plotting"
          n36 = mathscript code="width = 8;\nW = 32;\nlen = 88;\noffset=-10;\n% line 1\ny1_1 = [1.5:0.1:89.5];\ny1 = y1_1-offset;\nx1 = -width/2*ones(1,length(y1_1));\nk11 = 25/(W-width)*2;\ny11_1 = [(1.5):-0.1:(1.5-25)];\ny11 = y11_1 - offset;\nx11 = -width/2-((89.5-len)-y11_1)/k11;\n\n% line 2\ny2_1 = [1.5:0.1:89.5];\ny2 = y2_1 - offset;\nx2 = width/2*ones(1,length(y2_1));\nk22 = 28/(W-width)*2;\ny22_1 = [1.5:-0.1:(1.5-28)];\ny22 = y22_1-offset;\nx22 = width/2+((89.5-len)-y11_1)/k11;\n\n% line 3\ny3_1 = [(1.6-16):-0.1:(1.6-16-33.333)];\ny3 = y3_1-offset;\nx3 = -(1.6-16-y3_1)/k11;\n\n% line 4\ny4_1 = [(1.6-16):-0.1:(1.6-16-33.333)];\ny4 = y4_1-offset;\nx4 = (1.6-16-y4_1)/k11;"() -> ("y1"=w198:dbl[], "x1"=w197:dbl[], "y11"=w196:dbl[], "x11"=w195:dbl[], "y2"=w192:dbl[], "x2"=w191:dbl[], "y22"=w189:dbl[], "x22"=w188:dbl[], "y3"=w186:dbl[], "x3"=w185:dbl[], "y4"=w183:dbl[], "x4"=w182:dbl[])  [unwired: 1 in, 1 out]
          n37 = Bundle("y1"=w198, "x1"=w197) -> (w194:cluster{"y1":dbl[], "x1":dbl[]})  [unwired: 1 in]
          n38 = Bundle("y11"=w196, "x11"=w195) -> (w193:cluster{"y11":dbl[], "x11":dbl[]})  [unwired: 1 in]
          n39 = Bundle("y2"=w192, "x2"=w191) -> (w190:cluster{"y2":dbl[], "x2":dbl[]})  [unwired: 1 in]
          n40 = Bundle("y22"=w189, "x22"=w188) -> (w187:cluster{"y22":dbl[], "x22":dbl[]})  [unwired: 1 in]
          n41 = Bundle("y3"=w186, "x3"=w185) -> (w184:cluster{"y3":dbl[], "x3":dbl[]})  [unwired: 1 in]
          n42 = Bundle("y4"=w183, "x4"=w182) -> (w181:cluster{"y4":dbl[], "x4":dbl[]})  [unwired: 1 in]
          n43 = Build Array(w194, w193, w190, w187, w184, w181) -> (w180:cluster{"y4":dbl[], "x4":dbl[]}[])
        }
      }
      n44 = Initialize Array(0.0 ("element"), 0 ("dimension size")) -> (w26:dbl[])
      n45 = Initialize Array(0.0 ("element"), 0 ("dimension size")) -> (w25:dbl[])
      n46 = Initialize Array(0.0 ("element"), 48 ("dimension size")) -> (w34:dbl[])
    }
    frame #1 {
      # "Plotting"
      n47 = while {
        shift-right: [w3404] -> _
        shift-left: w991 -> [w3399]
        shift-right: [w3405] -> _
        shift-left: w992 -> [w3396]
        tunnel: w993 -> [w3401]
        tunnel: w991 -> [w3394]
        stop <- w3400 stop-if-true
        n48 = local read "Action Mode"() -> (w3402:T1)
        n49 = call "Wait"("Count(mSec)"=u32 250) -> ()  [unwired: 1 out]
        n50 = Select(t=w3394, s="Clear plot?", f=w3399) -> (s? t:f=w3398:dbl[])
        n51 = Select(t=w3394, s="Clear plot?", f=w3396) -> (s? t:f=w3395:dbl[])
        n52 = case shown="\"Sensing\", Default" w3402 {
          tunnel: w3398 -> [w3407 w3412 w3430]
          tunnel: w3395 -> [w3408 w3413 w3429]
          tunnel: [w3408 w3413 w3428] -> w3405
          tunnel: [w3407 w3412 w3427] -> w3404
          tunnel: [w3410 w3415 w3422] -> w3403
          tunnel: w3401 -> [w3409 w3414 w3417]
          frame "Actuation" {
            n53 = Bundle(w3408, w3407) -> (w3411:cluster{dbl[], dbl[]})  [unwired: 1 in]
            n54 = Build Array (concatenate)(w3411, w3409) -> (w3410:cluster{"y4":dbl[], "x4":cdb[]}[])
          }
          frame "Waiting" {
            n55 = Bundle(w3413, w3412) -> (w3416:cluster{dbl[], dbl[]})  [unwired: 1 in]
            n56 = Build Array (concatenate)(w3416, w3414) -> (w3415:cluster{"y4":dbl[], "x4":cdb[]}[])
          }
          frame "Sensing", Default {
            # "X"
            # "Y"
            n57 = local read "pm_hat_opt"() -> (w3420:dbl[])
            n58 = Index Array(array=w3420, index #1=0 ("index"), index #2=1 ("index")) -> (element #1=w3419:dbl, element #2=w3418:dbl)
            n59 = Multiply(x=1000.0, y=w3419) -> (x*y=w3423:dbl)
            n60 = Multiply(x=w3418, y=-1000.0) -> (x*y=w3425:dbl)
            n61 = Build Array (concatenate)(w3430, w3423) -> (w3427:dbl[])
            n62 = Build Array (concatenate)(w3429, w3425) -> (w3428:dbl[])
            n63 = Bundle(w3428, w3427) -> (w3421:cluster{dbl[], dbl[]})  [unwired: 1 in]
            n64 = Build Array (concatenate)(w3421, w3417) -> (w3422:cluster{"y4":dbl[], "x4":cdb[]}[])
          }
        }
        "XY Graph" <- w3403
        n65 = local read "stop"() -> (w3400:bool)
      }
      n66 = local read "Update M in realtime?"() -> (w988:bool)
      n67 = case shown="False" w988 {
        tunnel: [w998 w1010] -> w989
        tunnel: w990 -> [w1009 w1010]
        frame False {
          n68 = Index Array(array=w1009, index #1=0 ("index"), index #2=1 ("index"), index #3=2 ("index"), index #4=3 ("index"), index #5=4 ("index")) -> (element #1=w1003:dbl, element #2=w1002:dbl, element #3=w1001:dbl, element #4=w1000:dbl, element #5=w999:dbl)
          n69 = Build Array(w1003, w1002, w1001, w1000, w999) -> (w998:dbl[])
        }
        frame True {
        }
      }
      n70 = while {
        shift-right: [w1013] -> _
        shift-left: w997 -> [w1019]
        shift-right: [w1018] -> _
        shift-left: w989 -> [w1017]
        tunnel: w996 -> [w1016]
        tunnel: w995 -> [w1015]
        tunnel: w994 -> [w1014]
        stop <- "stop" stop-if-true
        n71 = case shown="\"Actuation\"" "Action Mode" {
          tunnel: w1019 -> [w1021 w1181 w1230]
          tunnel: [w1020 w1182 w1229] -> w1018
          tunnel: w1017 -> [w1020 w1182 w1228]
          tunnel: w1016 -> [_ _ w1227]
          tunnel: w1015 -> [_ _ w1226]
          tunnel: w1014 -> [_ _ w1225]
          tunnel: [w1021 w1181 w1224] -> w1013
          frame "Actuation" {
            n72 = flat-sequence {
              frame #0 {
                n73 = xnode "Analog input (1 sample) 3"() -> ("SteeringInput (C/AI1 (AI1))"=w1026:dbl)  [unwired: 1 in, 1 out]
                "Encoder 2" <- w1026
                n74 = call "Wait2"("Count(uSec)"=u32 1000 ("Count(mSec)")) -> ()  [unwired: 1 out]
                n75 = formula code="duty = 1-(input - min_v)/ (max_v-min_v);"("input"=w1026, "min_v"=3, "max_v"=10) -> ("duty"=w1025:dbl)
                n76 = xnode "Digital input (1 sample)"() -> ("Turning direction (C/DIO0 (DIO0))"=w1022:bool)  [unwired: 1 in, 1 out]
                n77 = Select(t=-1, s=w1022, f=1) -> (s? t:f=w1028:i32)
                n78 = Multiply(x=w1028, y=w1025) -> (x*y=w1027:dbl)
                n79 = Multiply(x="Steering gain", y=w1027) -> (x*y=w1031:dbl)
                "Duty Ratio" <- w1031
                n80 = Select(t=w1031, s="Actuation on?", f=0.0) -> (s? t:f=w1035:dbl)
                n81 = Absolute Value(x=w1035) -> (abs(x)=w1036:dbl)
                n82 = Greater Than 0?(x=w1035) -> (x > 0?=w1034:bool)
                n83 = xnode "PWM 2"("Duty Cycle"=w1036) -> ()  [unwired: 1 in, 1 out]
                n84 = xnode "Digital output (1 sample)"("C/DIO2 (DIO2)"=w1034) -> ()  [unwired: 1 in, 1 out]
              }
            }
          }
          frame "Waiting" {
            # "Change to next Sensing mode"
            # "Gradually decrease to zero"
            # "wait for field to disappear"
            n85 = flat-sequence {
              frame #0 {
                n86 = local write "Actuation on?"(FALSE ("Actuation on?")) -> ()
                n87 = call "Wait3"("Count(mSec)"=u32 60) -> ()  [unwired: 1 out]
                n88 = local read "Duty Ratio"() -> (w1183:dbl)
                n89 = xnode "PWM"("Duty Cycle"=w1183) -> ()  [unwired: 1 in, 1 out]
              }
            }
          }
          frame "Sensing", Default {
            n90 = call "Tick Count"() -> ("Tick Count(uSec)"=w1223:u32)
            n91 = flat-sequence {
              tunnel: [w1233] -> w1231
              tunnel: w1230 -> [w1232]
              tunnel: w1231 -> [w1472]
              tunnel: [w1477] -> w1229
              tunnel: w1228 -> [w1476]
              tunnel: w1227 -> [w1475]
              tunnel: w1226 -> [w1474]
              tunnel: w1225 -> [w1473]
              tunnel: [w1472] -> w1224
              frame #0 {
                # "Run 8 Iterations to read all sensors data simultaneously"
                n92 = for {
                  N: 8 -> [_]
                  shift-right: [w1246] -> w1233
                  shift-left: w1232 -> [w1248]
                  i -> [w1249]
                  # "B_meas"
                  n93 = Decrement(x=w1249) -> (x-1=w1242:i32)
                  n94 = Quotient & Remainder(x=w1242, y=8) -> (x-y*floor(x/y)=w1250:i32)  [unwired: 1 out]
                  n95 = Less Or Equal?(x=w1242, y=3) -> (x <= y?=w1240:bool)
                  n96 = Multiply(x=w1242, y=3) -> (x*y=w1239:i32)
                  n97 = Scale By Power Of 2(n=w1250, x=1) -> (x*2^n=w1251:i32)
                  n98 = Select(t=0, s=w1240, f=24) -> (s? t:f=w1236:i32)
                  n99 = Add(x=w1239, y=12) -> (x+y=w1243:i32)
                  n100 = Add(x=w1239, y=w1236) -> (x+y=w1235:i32)
                  n101 = Build Array(w1251) -> (w1253:i32[])
                  n102 = flat-sequence {
                    tunnel: w1253 -> [w1266]
                    tunnel: [w1266] -> w1256
                    tunnel: [w1264] -> w1255
                    tunnel: w1248 -> [w1260]
                    tunnel: [w1259] -> w1247
                    tunnel: w1243 -> [w1257]
                    tunnel: w1256 -> [w1373]
                    tunnel: w1255 -> [w1371]
                    tunnel: w1247 -> [w1370]
                    tunnel: [w1369] -> w1246
                    tunnel: w1235 -> [w1364]
                    frame #0 {
                      w1275 = i16 3000  # Gain Lsb/G
                      # "Sensor 5,6,7,8,9,10,11,12"
                      # "Z"
                      # "Y"
                      # "X"
                      n103 = xnode "I2C Multiplex 2"("Slave Address (7-bit)"=u8 112, "Bytes to Write"=w1266) -> ("error out"=w1265:errorcluster)  [unwired: 1 in]
                      n104 = Build Array(u8 0) -> (w1279:u8[])
                      n105 = xnode "I2C 2"("Slave Address (7-bit)"=u8 13, "Bytes to Write"=w1279, "Byte Count"=u32 6, "error in (no error)"=w1265) -> ("Bytes Read"=w1282:u8[], "error out"=w1264:errorcluster)
                      n106 = Index Array(array=w1282) -> (element #1=w1274:u8, element #2=w1273:u8, element #3=w1271:u8, element #4=w1272:u8, element #5=w1269:u8, element #6=w1270:u8)  [unwired: 6 in]
                      n107 = Join Numbers(hi=w1273, lo=w1274) -> ((hi.lo)=w1285:u16)
                      n108 = Join Numbers(hi=w1272, lo=w1271) -> ((hi.lo)=w1283:u16)
                      n109 = Join Numbers(hi=w1270, lo=w1269) -> ((hi.lo)=w1284:u16)
                      n110 = To Word Integer(number=w1285) -> (16bit integer=w1278:i16)
                      n111 = To Word Integer(number=w1283) -> (16bit integer=w1277:i16)
                      n112 = To Word Integer(number=w1284) -> (16bit integer=w1276:i16)
                      n113 = Divide(x=w1278, y=w1275) -> (x/y=w1263:dbl)
                      n114 = Divide(x=w1277, y=w1275) -> (x/y=w1262:dbl)
                      n115 = Divide(x=w1276, y=w1275) -> (x/y=w1261:dbl)
                      n116 = Build Array(w1263, w1262, w1261) -> (w1258:dbl[])
                      n117 = Replace Array Subset(array=w1260, new element=w1258, index=w1257) -> (w1259:dbl[])
                    }
                    frame #1 {
                      w1382 = i16 3000  # Gain Lsb/G
                      # "Sensor 1,2,3,4,13,14,15,16"
                      n118 = xnode "I2C Multiplex 3"("Slave Address (7-bit)"=u8 113, "Bytes to Write"=w1373, "error in (no error)"=w1371) -> ("error out"=w1372:errorcluster)
                      n119 = Build Array(u8 0) -> (w1386:u8[])
                      n120 = xnode "I2C"("Slave Address (7-bit)"=u8 13, "Bytes to Write"=w1386, "Byte Count"=u32 6, "error in (no error)"=w1372) -> ("Bytes Read"=w1389:u8[])  [unwired: 1 out]
                      n121 = Index Array(array=w1389) -> (element #1=w1381:u8, element #2=w1380:u8, element #3=w1378:u8, element #4=w1379:u8, element #5=w1376:u8, element #6=w1377:u8)  [unwired: 6 in]
                      n122 = Join Numbers(hi=w1380, lo=w1381) -> ((hi.lo)=w1392:u16)
                      n123 = Join Numbers(hi=w1379, lo=w1378) -> ((hi.lo)=w1390:u16)
                      n124 = Join Numbers(hi=w1377, lo=w1376) -> ((hi.lo)=w1391:u16)
                      n125 = To Word Integer(number=w1392) -> (16bit integer=w1385:i16)
                      n126 = To Word Integer(number=w1390) -> (16bit integer=w1384:i16)
                      n127 = To Word Integer(number=w1391) -> (16bit integer=w1383:i16)
                      n128 = Divide(x=w1385, y=w1382) -> (x/y=w1368:dbl)
                      n129 = Divide(x=w1384, y=w1382) -> (x/y=w1367:dbl)
                      n130 = Divide(x=w1383, y=w1382) -> (x/y=w1366:dbl)
                      n131 = Build Array(w1368, w1367, w1366) -> (w1365:dbl[])
                      n132 = Replace Array Subset(array=w1370, new element=w1365, index=w1364) -> (w1369:dbl[])
                    }
                  }
                }
              }
              frame #1 {
                # "B_earth_field"
                n133 = Subtract(x=w1472, y=w1473) -> (x-y=w1478:dbl[])
                n134 = case shown="False" "Update M in realtime?" {
                  tunnel: w1478 -> [w1483 w2447]
                  tunnel: [w1479 w2446] -> w1477
                  tunnel: w1476 -> [w1480 w2445]
                  tunnel: w1475 -> [w1481 w2444]
                  tunnel: w1474 -> [w1482 w2443]
                  frame False {
                    n135 = mathscript code="pm_init = pm_init';\ny_meas = y_meas*1e-4;  % convert from Gauss to Tesla\nn_par = length(pm_init);\niteration = 0;  % current number of \nstop = 0;  % stop flag\nMaxIter = 100;   % maximum number of iteration\nepsilon_1 = 1e-10;  % convergence tolerance for gradient\nepsilon_2 = 1e-9;  % convergence tolerance for parameter\nepsilon_3 = 1e-15;  % convergence tolerance for residual error\nepsilon_4 = 1e-8;  % determines acceptance of a L-M step\npm = pm_init; % initialization on parameters\nlambda_0 = 1e-3;  % user-specified initial lambda\n% Jacobian initialization\nJ = Analytic_Jacobian_Mag_cir_array_noM(pm_init,xyz_s,meas_dir_s,M);\n% initialize L-M parameters\nlambda = lambda_0*max(diag(J'*J));\nv = 2;  % scale factor\nwhile ( ~stop)\n    iteration = iteration + 1;\n    B_meas = PM_forward_field_noM(pm,xyz_s,meas_dir_s,M);\n% compute residual error between model and measurement\n    err = (y_meas - B_meas)';\n    if ( norm(err)^2< epsilon_3 &&  iteration > 2 )\n        stop = 1;\n        break;\n    end\n    % compute gradient\n    grad = J'*err;\n    % check stopping criterion 1\n    if ( max(abs(grad)) < epsilon_1  &&  iteration > 2 )\n        stop = 1;\n        break\n    end\n    % parameter increment change\n    delta = (J'*J + lambda*eye(n_par))\\J'*err;  % simplest version\n    % check stopping criterion 2 \n    if ( max(abs(delta)./(abs(pm)+1e-20)) < epsilon_2  &&  iteration > 2 )\n        stop = 1;\n        break\n    end\n    pm_try = pm + delta;\n    % evaluate value using pm_try\n    B_meas_try = PM_forward_field_noM(pm_try,xyz_s,meas_dir_s,M);  % compute measurement based on given direction\n    err_try = (y_meas - B_meas_try)';\n    % compute rho for determining acceptance\n    rho = (err'*err - err_try'*err_try)/(delta'*(lambda*delta + J'*err) );\n    if rho > epsilon_4   % if better\n        pm = pm_try;  % accpet pm_try\n        lambda = lambda*max( 1/3, 1-(2*rho-1)^3 );\n        v = 2;\n             % update Jacobian matrix\n        J = Analytic_Jacobian_Mag_cir_array_noM(pm,xyz_s,meas_dir_s,M);\n    else      % if not better\n        lambda = lambda*v;\n        v = 2*v;\n    end\n    if ( iteration == MaxIter )\n        stop = 1;\n    end\nend\n\npm_hat_opt = pm;"("meas_dir_s"=w1482, "xyz_s"=w1481, "y_meas"=w1483, "pm_init"=w1480, "M"="M") -> ("pm_hat_opt"=w1479:dbl[])  [unwired: 1 in, 1 out]
                  }
                  frame True {
                    # "Use current optimal point as initial guess for next iteration"
                    n136 = mathscript code="pm_init = pm_init';\ny_meas = y_meas*1e-4;  % convert from Gauss to Tesla\nn_par = length(pm_init);\niteration = 0;  % current number of \nstop = 0;  % stop flag\nMaxIter = 100;   % maximum number of iteration\nepsilon_1 = 1e-10;  % convergence tolerance for gradient\nepsilon_2 = 1e-9;  % convergence tolerance for parameter\nepsilon_3 = 1e-15;  % convergence tolerance for residual error\nepsilon_4 = 1e-8;  % determines acceptance of a L-M step\npm = pm_init; % initialization on parameters\nlambda_0 = 1e-3;  % user-specified initial lambda\n% Jacobian initialization\nJ = Analytic_Jacobian_Mag_cir_array_test(pm_init,xyz_s,meas_dir_s);\n% initialize L-M parameters\nlambda = lambda_0*max(diag(J'*J));\nv = 2;  % scale factor\nwhile ( ~stop)\n    iteration = iteration + 1;\n    B_meas = PM_forward_field(pm,xyz_s,meas_dir_s);\n% compute residual error between model and measurement\n    err = (y_meas - B_meas)';\n    if ( norm(err)^2< epsilon_3 &&  iteration > 2 )\n        stop = 1;\n        break;\n    end\n    % compute gradient\n    grad = J'*err;\n    % check stopping criterion 1\n    if ( max(abs(grad)) < epsilon_1  &&  iteration > 2 )\n        stop = 1;\n        break\n    end\n    % parameter increment change\n    delta = (J'*J + lambda*eye(n_par))\\J'*err;  % simplest version\n    % check stopping criterion 2 \n    if ( max(abs(delta)./(abs(pm)+1e-20)) < epsilon_2  &&  iteration > 2 )\n        stop = 1;\n        break\n    end\n    pm_try = pm + delta;\n    % evaluate value using pm_try\n    B_meas_try = PM_forward_field(pm_try,xyz_s,meas_dir_s);  % compute measurement based on given direction\n    err_try = (y_meas - B_meas_try)';\n    % compute rho for determining acceptance\n    rho = (err'*err - err_try'*err_try)/(delta'*(lambda*delta + J'*err) );\n    if rho > epsilon_4   % if better\n        pm = pm_try;  % accpet pm_try\n        lambda = lambda*max( 1/3, 1-(2*rho-1)^3 );\n        v = 2;\n             % update Jacobian matrix\n        J = Analytic_Jacobian_Mag_cir_array_test(pm,xyz_s,meas_dir_s);\n    else      % if not better\n        lambda = lambda*v;\n        v = 2*v;\n    end\n    if ( iteration == MaxIter )\n        stop = 1;\n    end\nend\n\npm_hat_opt = pm;"("meas_dir_s"=w2443, "xyz_s"=w2444, "y_meas"=w2447, "pm_init"=w2445) -> ("pm_hat_opt"=w2446:dbl[])  [unwired: 1 in, 1 out]
                  }
                }
                "pm_hat_opt" <- w1477
              }
            }
            n137 = feedback #1() -> (w1222:u32)  [unwired: 1 in]
            n138 = feedback-in #1(w1223) -> ()
            n139 = Subtract(x=w1223, y=w1222) -> (x-y=→"Sensing time":u32)
          }
        }
      }
    }
    frame #2 {
      n140 = xnode "PWM 3"("Duty Cycle"=0.0) -> ()  [unwired: 1 in, 1 out]
    }
  }
